vi "与工控机交互(子VI).vi"   [LabVIEW 2016, in "数据传输系统.lvlib"]
types:
  T1 = cluster{"setini":string, "sysini":string, "hechaini":string, "actualwrite":string, "actualread":string, "datasent":string, "反控命令信息队列":string, "反控与仪器交互":string}
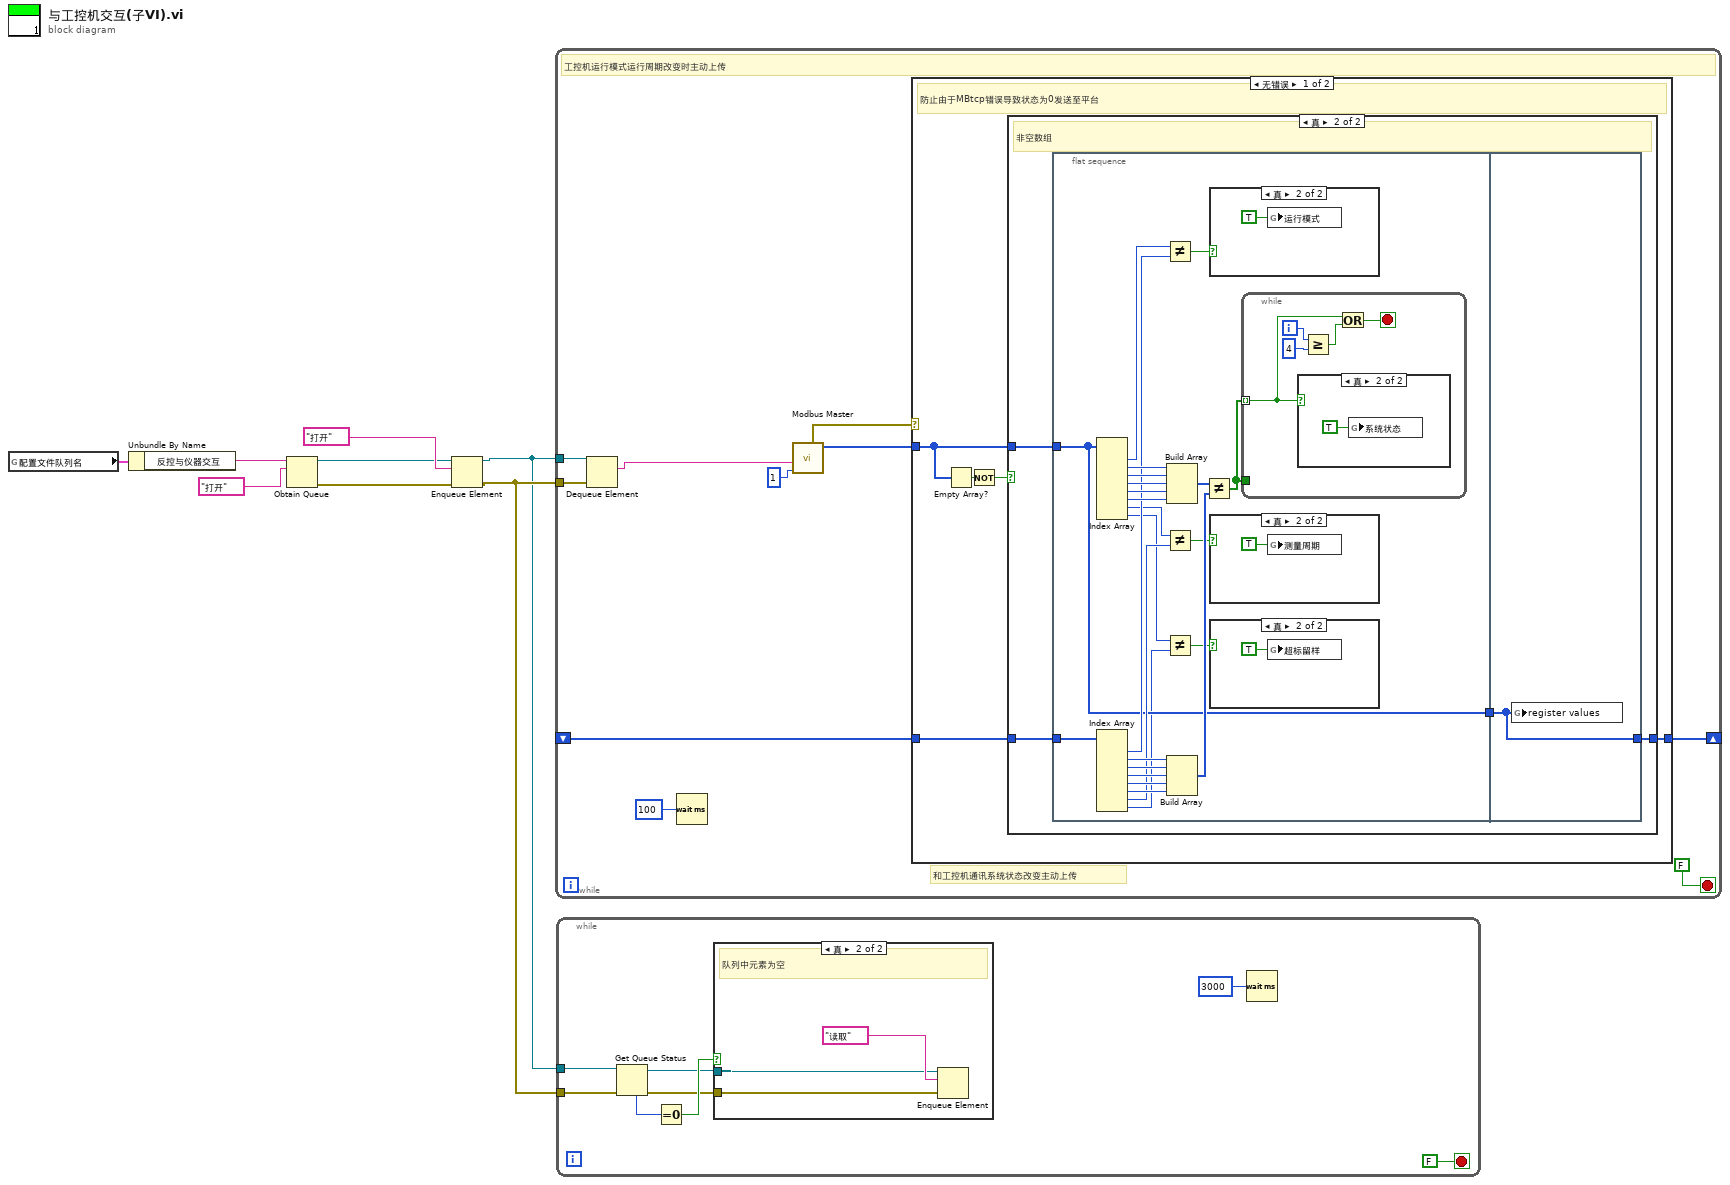
[diagram p0: block diagram]
diagram:
  n1 = global read "断电保存全局.vi" "配置文件队列名"() -> (w2:T1)
  n2 = Unbundle By Name(w2) -> ("反控与仪器交互"=w1:string)
  n3 = Obtain Queue(name (unnamed)=w1, element data type="打开" ("读取写入选择")) -> (queue out=w4:refnum<queue>, error out=w5:errorcluster)  [unwired: 3 in, 1 out]
  n4 = Enqueue Element(queue=w4, element="打开" ("读取写入选择"), error in (no error)=w5) -> (queue out=w6:refnum<queue>, error out=w7:errorcluster)  [unwired: 1 in, 1 out]
  n5 = while {
    tunnel: w6 -> [w13]
    tunnel: w7 -> [w12]
    shift-right: [w9] -> _
    shift-left: _ -> [w10]
    stop <- FALSE stop-if-true
    # "和工控机通讯系统状态改变主动上传"
    # "工控机运行模式运行周期改变时主动上传"
    n6 = Dequeue Element(queue=w13, error in (no error)=w12) -> (element=w11:string)  [unwired: 1 in, 3 out]
    n7 = Wait (ms)(milliseconds to wait=u32 100 ("等待时间（毫秒）")) -> ()  [unwired: 1 out]
    n8 = call "Modbus Master.vi"("Unit ID"=u8 1, "读取写入选择"=w11) -> ("register values"=w16:u16[], "error out"=w15:errorcluster)  [unwired: 8 in]
    n9 = case shown="无错误" w15 {
      tunnel: w16 -> [w21 _]
      tunnel: w10 -> [w23 w63]
      tunnel: [w22 w63] -> w9
      frame No Error {
        # "防止由于MBtcp错误导致状态为0发送至平台"
        n10 = Empty Array?(array=w21) -> (empty?=w20:bool)
        n11 = Not(x=w20) -> (.not. x?=w19:bool)
        n12 = case shown="真" w19 {
          tunnel: w23 -> [w24 w27]
          tunnel: [w24 w26] -> w22
          tunnel: w21 -> [_ w25]
          frame False {
          }
          frame True {
            # "非空数组"
            n13 = flat-sequence {
              tunnel: w25 -> [w34]
              tunnel: [w34] -> w28
              tunnel: w27 -> [w30]
              tunnel: w28 -> [w62]
              tunnel: [w62] -> w26
              frame #0 {
                n14 = Index Array(array=w34) -> (element #1=w40:u16, element #2=w52:u16, element #3=w51:u16, element #4=w50:u16, element #5=w49:u16, element #6=w48:u16, element #7=w38:u16, element #8=w33:u16)  [unwired: 8 in]
                n15 = Index Array(array=w30) -> (element #1=w39:u16, element #2=w47:u16, element #3=w46:u16, element #4=w45:u16, element #5=w44:u16, element #6=w43:u16, element #7=w37:u16, element #8=w32:u16)  [unwired: 8 in]
                n16 = Not Equal?(x=w40, y=w39) -> (x != y?=w35:bool)
                n17 = Not Equal?(x=w38, y=w37) -> (x != y?=w36:bool)
                n18 = Not Equal?(x=w33, y=w32) -> (x != y?=w31:bool)
                n19 = Build Array(w52, w51, w50, w49, w48) -> (w42:u16[])
                n20 = Build Array(w47, w46, w45, w44, w43) -> (w41:u16[])
                n21 = Not Equal?(x=w42, y=w41) -> (x != y?=w29:bool[])
                n22 = case shown="真" w35 {
                  frame False {
                  }
                  frame True {
                    n23 = global write "全局1.vi" "运行模式"(TRUE) -> ()
                  }
                }
                n24 = case shown="真" w36 {
                  frame False {
                  }
                  frame True {
                    n25 = global write "全局1.vi" "测量周期"(TRUE ("系统状态改变")) -> ()
                  }
                }
                n26 = case shown="真" w31 {
                  frame False {
                  }
                  frame True {
                    n27 = global write "全局1.vi" "超标留样"(TRUE ("系统状态改变")) -> ()
                  }
                }
                n28 = while {
                  tunnel: w29 -> [w56] mode=indexing
                  tunnel: w29 -> [_]
                  i -> [w58]
                  stop <- w54 stop-if-true
                  n29 = case shown="真" w56 {
                    frame False {
                    }
                    frame True {
                      n30 = global write "全局1.vi" "系统状态"(TRUE ("系统状态改变")) -> ()
                    }
                  }
                  n31 = Greater Or Equal?(x=w58, y=4) -> (x >= y?=w55:bool)
                  n32 = Or(x=w56, y=w55) -> (x .or. y?=w54:bool)
                }
              }
              frame #1 {
                n33 = global write "全局1.vi" "register values"(w62) -> ()
              }
            }
          }
        }
      }
      frame Error {
      }
    }
  }
  n34 = while {
    tunnel: w6 -> [w68]
    tunnel: w7 -> [w67]
    stop <- FALSE stop-if-true
    n35 = Get Queue Status(queue=w68, error in (no error)=w67) -> (queue out=w65:refnum<queue>, error out=w64:errorcluster, # elements in queue=w69:i32)  [unwired: 1 in, 5 out]
    n36 = Equal To 0?(x=w69) -> (x = 0?=w66:bool)
    n37 = case shown="真" w66 {
      tunnel: w65 -> [_ w73]
      tunnel: w64 -> [_ w72]
      frame False {
      }
      frame True {
        # "队列中元素为空"
        n38 = Enqueue Element(queue=w73, element="读取" ("读取写入选择"), error in (no error)=w72) -> ()  [unwired: 1 in, 3 out]
      }
    }
    n39 = Wait (ms)(milliseconds to wait=u32 3000 ("等待时间（毫秒）")) -> ()  [unwired: 1 out]
  }
